vi "MoveAxis.vi"(8 "error in (no error)":errorcluster, 9 "Position":u16, 10 "Axis":T1, 11 "MotorController in":refnum<class "MotorController.lvclass">) -> (0 "error out":errorcluster, 3 "MotorController out":refnum<class "MotorController.lvclass">)   [LabVIEW 2019, in "MotorController.lvclass"]
uses:
  MotorController.lvclass
  Axes_enum_typedef.ctl
  MotorController.lvclass/MotorController.ctl
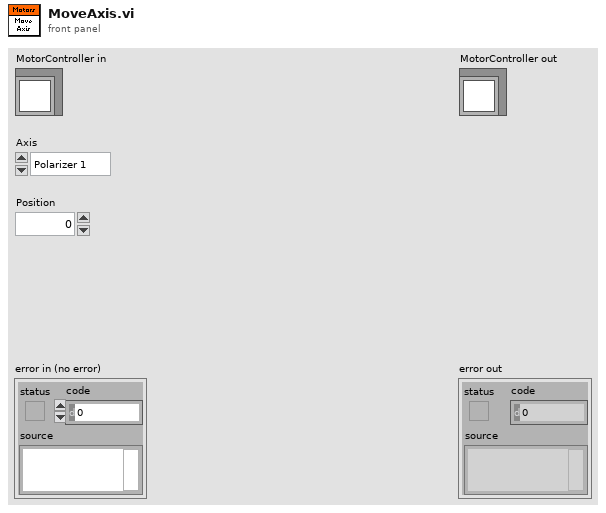
[diagram p1: front panel]
types:
  T1 = typedef "Axes_enum_typedef.ctl" = enum16{"Polarizer 1", "Polarizer 2", "Sample", "Stage"}
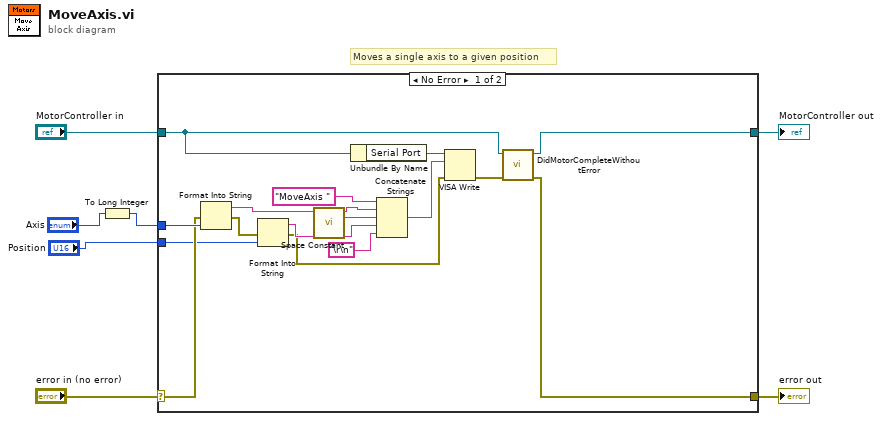
[diagram p0: block diagram]
diagram:
  # "Moves a single axis to a given position"
  n1 = To Long Integer(number="Axis") -> (32bit integer=w1:i32)
  n2 = case shown="No Error" "error in (no error)" {
    selector: "error in (no error)" -> [w19 w25]
    tunnel: [w8 w25] -> w6
    tunnel: [w9 w24] -> w4
    tunnel: "MotorController in" -> [w11 w24]
    tunnel: w1 -> [w21 _]
    tunnel: "Position" -> [w18 _]
    frame No Error {
      n3 = Format Into String(error in=w19, w21) -> (resulting string=w17:string, error out=w20:errorcluster)  [unwired: 2 in]
      n4 = Format Into String(error in=w20, w18) -> (resulting string=w15:string, error out=w13:errorcluster)  [unwired: 2 in]
      n5 = call <vilib>:"Space Constant.vi"() -> ("String"=w16:string)
      n6 = Unbundle By Name(w11) -> ("Serial Port"=w23:refnum<visa-resource-name>)
      n7 = Concatenate Strings("MoveAxis ", w17, w16, w15, "\r\n") -> (w12:string)
      n8 = VISA Write(VISA resource name=w23, write buffer=w12, error in (no error)=w13) -> (error out=w10:errorcluster)  [unwired: 2 out]
      n9 = call "DidMotorCompleteWithoutError.vi"("error in (no error)"=w10, "MotorController in"=w11) -> ("error out"=w8:errorcluster, "MotorController out"=w9:refnum<class "MotorController.lvclass">)  [unwired: 7 in, 1 out]
    }
    frame Error {
    }
  }
  "error out" <- w6
  "MotorController out" <- w4
